vi "Main.vi"(7 "sweep rate, /min":dbl=0.2, 8 "sweep to:":dbl=4.0, 9 "sweep":T8(radio)=enum."2636a_smub") -> ()   [LabVIEW 2021]
uses:
  controls/Channel.ctl
  <instrlib>/Zurich Instruments LabOne/Public/ziTypeHandle.ctl
  controls/Measure.ctl
  controls/iPSreadCtrl.ctl
  controls/iTCreadCtrl.ctl
  controls/iPSsetCtrl.ctl
  subVIs/MFLIcommand.ctl
  controls/Source.ctl
  controls/iTCsetCtrl.ctl
  <vilib>/Utility/file.llb/Write To Spreadsheet File (DBL).vi
  <vilib>/gmath/NI_Gmath.lvlib
  <instrlib>/Keithley 2450/Keithley 2450.lvlib
  HULK SMS/SMScontrols.ctl
  <instrlib>/Zurich Instruments LabOne/Zurich Instruments LabOne.lvlib
panel:
  in  "MFLI1_AuxOut0":bool
  in  "T_Channel_sweep":i32=8
  in  "MC_RuO2":bool
  out "HandleOut 4":T1 {"Handle" format="0x%08x"; "Conn" format="0x%08x"}
  out "HandleOut 3":T1 {"Handle" format="0x%08x"; "Conn" format="0x%08x"}
  out "HandleOut 2":T1 {"Handle" format="0x%08x"; "Conn" format="0x%08x"}
  in  "MFLI4_d3":bool
  in  "MFLI4_d2":bool
  in  "MFLI4_d1":bool
  in  "MFLI4_d0":bool=TRUE
  in  "MFLI4_addr":string="DEV3532"
  in  "MFLI3_d3":bool
  in  "MFLI3_d2":bool
  in  "MFLI3_d1":bool
  in  "MFLI3_d0":bool=TRUE
  in  "MFLI3_addr":string="DEV3550"
  in  "MFLI2_d3":bool
  in  "MFLI2_d2":bool
  in  "MFLI2_d1":bool
  in  "MFLI2_d0":bool=TRUE
  in  "MFLI2_addr":string="DEV4330"
  in  "MFLI1_d3":bool
  in  "MFLI1_d2":bool
  out "HandleOut":T1 {"Handle" format="0x%08x"; "Conn" format="0x%08x"}
  in  "MFLI1_d1":bool
  in  "MFLI1_d0":bool=TRUE
  in  "MFLI1_addr":string="DEV4406"
  in  "SR830 5 oop":bool
  in  "SR830 5 ip":bool
  in  "SR830 5 addr":u8=5
  in  "SR830 4 oop":bool
  in  "SR830 4 ip":bool
  in  "SR830 3 oop":bool
  in  "SR830 3 ip":bool
  in  "SR830 2 oop":bool
  in  "SR830 2 ip":bool
  in  "SR830 1 oop":bool
  in  "SR830 1 ip":bool
  in  "SR830 4 addr":u8=4
  in  "SR830 3 addr":u8=3
  in  "SR830 2 addr":u8=2
  in  "SR830 1 addr":u8=1
  in  "MC_Cernox":bool
  in  "PT2":bool
  in  "Still":bool
  in  "Cold_Plate":bool
  in  "PT1":bool
  in  "Magnet_T":bool
  in  "2182A 4 ch2":bool
  in  "2182A 4 ch1":bool
  in  "2182A 3 ch2":bool
  in  "2182A 3 ch1":bool
  in  "2182A 2 ch2":bool
  in  "2182A 2 ch1":bool
  in  "2182A 4 addr":u8=18
  in  "2182A 3 addr":u8=17
  in  "2182A 2 addr":u8=16
  in  "2182A 1 addr":u8=15
  in  "2182A 1 ch2":bool
  in  "2182A 1 ch1":bool
  in  "Lead Chanl":T2(ring)=enum."time_sweep"
  in  "Sweep Up":bool
  in  "Stop Ramp":bool
  in  "Up Rate":dbl=0.2
  in  "Down Rate":dbl=0.2
  in  "Ramp \nUp":bool
  in  "Ramp\n Down":bool
  in  "lower limit":dbl=-4.0
  in  "upper limit":dbl=4.0
  in  "Sweep Down":bool
  in  "Stop Sweep":bool
  in  "Continuous Sweep":bool
  in  "Slave Chanl":T3=enum."b"
  in  "Double Sweep":bool
  in  "Slope":dbl
  in  "Offset":dbl
  in  "time/point, sec":dbl=1.0
  out "sweep value":dbl=2.186666666666735
  out "time delay, ms":dbl
  out "current time":timestamp=timestamp(3589630313.018 s since 1904-01-01) format="%<%H:%M:%S%1u>T"
  in  "Sweep B":bool
  out "SuperHyper":dbl=-0.4901
  in  "2461_addr_sweep":refnum<visa-resource-name>="itcetherT"
  in  "2461_meas_i":bool
  in  "2461_meas_v":bool
  out "Hyper Channel":dbl=-0.4901
  out "Sweep Channel":dbl
  out "Step Channel":dbl=-0.4901
  in  "MappingName":string
  in  "Data Folder":path=path "E:/Katya"
  out "Data file:":path=path "D:/Yanmeng/Data/Year2018/January2018/Jan2318/Jan2318x001.dat"
  in  "Initialize":bool=TRUE
  in  "Quit":bool
  in  "Refresh Time(ms)":u32=100
  in  "Monitor":bool
  in  "Linetrace or Mapping?":bool
  in  "Step and Hyerloop Setups":enum32{"Step", "HyperLoop", "SuperHyper"}(tab)
  in  "T_Channel":i32=8
  in  "Lead Chanl_step":T4(ring)=enum."2636a_smua_step" caption="Lead Chanl"
  in  "UpLimitValue":dbl
  in  "DownLimitValue":dbl
  in  "Change Sweep Range":bool
  in  "Offset_Up":dbl
  in  "Offset_Down":dbl
  in  "Slope":dbl
  in  "Down          Up":string[][](table)
  in  "Generate":bool
  in  "2461_addr_step":refnum<visa-resource-name>="itcetherT"
  in  "Channel":T3=enum."b"
  in  "Mini steps":dbl=30.0
  in  "Tolerance_Step":dbl=0.0001
  in  "Step Slope":dbl
  in  "Step Offset":dbl
  in  "diagonal step":bool
  in  "FieldRate(T/min)":dbl=0.001
  out "at field":bool
  in  "iPS _addr_step":refnum<visa-resource-name>="iPS"
  in  "step":T5(radio)=enum."time_step"
  in  "2614A_addr_step":refnum<visa-resource-name>="Keithley2614B"
  in  "2400_2_addr_step":u8=12
  in  "2400_1_addr_step":u8=12
  in  "wait between sweeps(s)":u32=1
  in  "Wait Between Step(s)":i32=1
  in  "Stop Mapping":bool
  in  "Start Mapping":bool
  in  "HyperLoop":bool
  in  "EstimateTime":bool
  out "MM:":dbl
  out "SS:":dbl
  out "HH:":dbl
  out "Finish Time":timestamp
  out "Sweep Direction":string
  out "Current Step Value":dbl
  out "Table Index":dbl
  in  "Populate step table?":bool
  in  "Step values":string[][](table)=[["-20"], ["-10"], ["-4"], ["-1"], ["3"], ["6"], ["10"], [""]]
  in  "to":dbl=1.0
  in  "step":dbl=0.001
  in  "from":dbl
  in  "SwapStepDirection":bool
  out "Hidden_HyperLoop_Swap":bool
  out "HyperLoop Hidden":bool
  in  "EstimateTime Hyper":bool
  out "MM:":dbl
  out "SS:":dbl
  out "HH:":dbl
  out "Finish Time 2":timestamp
  out "Sweep Direction 2":string
  out "Current Hyper Value":dbl
  out "HyperLoop Index":dbl
  in  "Populate HyperLoop table?":bool
  in  "HyperLoop Steps":string[][](table)=[["-20"], ["-10"], ["-4"], ["-1"], ["3"], ["6"], ["10"], [""]]
  in  "to":dbl=1.0
  in  "step":dbl=2.0
  in  "from":dbl=1.0
  in  "SuperHyper":bool
  in  "Channel_hyper":T3=enum."b"
  in  "Hyper_Mini steps":dbl=30.0
  in  "Tolerance_Hyper":dbl=0.1
  in  "Hyper Slope":dbl
  in  "Hyper Offset":dbl
  in  "diagonal_hyper":bool
  in  "Hyper_FieldRate\n(T/min)":dbl=0.1
  out "at field_hyper":bool
  in  "iPS _addr_hyper":refnum<visa-resource-name>="iPS"
  in  "iTC_addr_hyper":refnum<visa-resource-name>="iTC"
  in  "step_hyper":T6(radio)=enum."time_HyperLoop"
  in  "2336A_addr_hyper":refnum<visa-resource-name>="Keithley2614B"
  in  "2400_2_addr_hyper":u8=12
  in  "2400_1_addr_hyper":u8=12
  in  "Wait Between Hyper":i32=10
  in  "Stop HyperLoop":bool
  in  "Start HyperLoop":bool
  in  "SwapHyperDirection":bool
  out "Hidden_super_Swap":bool
  out "Super Hidden":bool
  in  "EstimateTime Hyper 2":bool
  out "MM:":dbl
  out "SS:":dbl
  out "HH:":dbl
  out "Finish Time Super":timestamp
  out "Sweep Direction3":string
  out "Current SuperHyper Value":dbl
  out "SuperHyper_Index":dbl
  in  "Populate SuperHyper table?":bool
  in  "SuperHyper Steps":string[][](table)=[["-20"], ["-10"], ["-4"], ["-1"], ["3"], ["6"], ["10"], [""]]
  in  "to":dbl=1.0
  in  "step":dbl=2.0
  in  "from":dbl=1.0
  in  "Channel_super":T3=enum."b"
  in  "Super_ministeps":dbl=30.0
  in  "Tolerance_super":dbl=0.1
  in  "Slope_super":dbl
  in  "Offset_super":dbl
  in  "diagona_super":bool
  in  "Super_FieldRate\n(T/min)":dbl=0.1
  out "at field_super":bool
  in  "iPS _addr_superhyper":refnum<visa-resource-name>="iPS"
  in  "iTC_addr_super":refnum<visa-resource-name>="iTC"
  in  "step_super":T7(radio)=enum."time_SuperHyper"
  in  "2336A_addr_super":refnum<visa-resource-name>="Keithley2614B"
  in  "2400_2_addr_super":u8=12
  in  "2400_1_addr_super":u8=12
  in  "Wait Btwn SuperHyper":i32=10
  in  "Stop SuperHyper":bool
  in  "StartSuperHyper":bool
  out "DownNameString":string
  out "UpNameString":string
  in  "Cytec_Switch":bool
  in  "Lockin_Setup":bool
  in  "TempCtrl":bool
  in  "MagnetCtrl":bool
  in  "Tolerance_Sweep":dbl=0.01
  in  "iPS_addr_sweep":refnum<visa-resource-name>="iPS"
  in  "2400 3 addr":u8=14
  in  "2400 2 addr":u8=12
  in  "2400 1 addr":u8=13
  in  "2614A addr":refnum<visa-resource-name>="TCPIP0::192.168.0.13::inst0::INSTR"
  in  "sweep":bool
  in  "MagnetField":bool
  in  "auto\nrange B":bool
  in  "measure time":bool
  in  "2636A smub meas i":bool=TRUE
  in  "2636A smub meas v":bool=TRUE
  in  "2636A smua meas i":bool
  in  "2636A smua meas v":bool
  in  "2400 3 meas i":bool
  in  "2400 2 meas i":bool
  in  "2400 2 meas v":bool
  in  "2400 3 meas v":bool
  in  "2400 1 meas i":bool
  in  "2400 1 meas v":bool
  in  "auto\nrange A":bool
  out "status 3":bool
  in  "Y_right_formula":string="brty/10/(300*10^-9)"
  in  "Yright":u16(ring)=3 caption="Y-Right:" items=["V_Sweep_AuxOut0", "2614A_smub_v", "2614A_smub_i", "time", "Magnet_Temp", "MC_RuO2_Temp", "MC_Cernox_Temp", "iTC_Step", "MFLI1_d0_x", "MFLI1_d0_y", "MFLI1_d0_freq", "MFLI1_d2_x", "MFLI1_d2_y", "MFLI1_d2_freq", "MF1_AuxOut0", "formula"]
  out "status 2":bool
  in  "Y_left_formula":string="brty/10/(300*10^-9)"
  in  "X_axis_formula":string
  in  "Yaxis":u16(ring)=3 caption="Y-Left:" items=["V_Sweep_AuxOut0", "2614A_smub_v", "2614A_smub_i", "time", "Magnet_Temp", "MC_RuO2_Temp", "MC_Cernox_Temp", "iTC_Step", "MFLI1_d0_x", "MFLI1_d0_y", "MFLI1_d0_freq", "MFLI1_d2_x", "MFLI1_d2_y", "MFLI1_d2_freq", "MF1_AuxOut0", "formula"]
  out "XY Graph":cluster{"Y Values":dbl[], "Y Values":dbl[]}[](graph)
  in  "Xaxis":u16(ring) caption="X-axis:" items=["V_Sweep_AuxOut0", "2614A_smub_v", "2614A_smub_i", "time", "Magnet_Temp", "MC_RuO2_Temp", "MC_Cernox_Temp", "iTC_Step", "MFLI1_d0_x", "MFLI1_d0_y", "MFLI1_d0_freq", "MFLI1_d2_x", "MFLI1_d2_y", "MFLI1_d2_freq", "MF1_AuxOut0", "formula"]
  out "status":bool
  in  "Show cursor":bool
  in  "Hulk_B_meas (Vnano)":bool
  in  "Hulk_SMS_addr":refnum<visa-resource-name>="TCPIP0::10.99.75.17::inst0::INSTR"
  in  "formula_variables":string[](array[string])=["a", "b", "c", "d", "e", "e", "f", "g", "h", "i", "j"]
  out "data":dbl[](array[numeric])
  out "Figure_axis":string[](array[string])=["HULK_SMS_output", "SR830_1_ip", "SR830_1_oop"]
  out "data_caption":string="HULK_SMS_output\tSR830_1_ip\tSR830_1_oop\t"
  # "Current Value of Sweep and Step Channels"
  # "Sweep Channel Setup"
  # "SweepChannel"
  # "address"
  # "2400_1"
  # "2400_2"
  # "2400_3"
  # "2614A_smua"
  # "2614A_smub"
  # "time"
  # "Triton B"
  # "MC_Temp"
  # "2450_1"
  # "MF1 AuxOut0"
  # "sweep"
  # "!Current sweep!"
  # "MagnetField"
  # "measure"
  # "voltage (_v)"
  # "current (_i)"
  # "blue"
  # "red"
  # "Measure Channels"
  # "MFLI Lock-in amplifiers"
  # "SRS Lock-in amplifiers"
  # "address"
  # "SR830_1"
  # "SR830_2"
  # "SR830_3"
  # "SR830_4"
  # "d0"
  # "measure"
  # "SR830_5"
  # "d1"
  # "in phase (_ip)"
  # "d2"
  # "out of phase (_oop)"
  # "d3"
  # "Nanovoltmeters"
  # "Temperature"
  # "address"
  # "Dilution Circuit"
  # "PulseTube"
  # "MC_RuO2"
  # "measure"
  # "2182A_1"
  # "2182A_2"
  # "2182A_3"
  # "2182A_4"
  # "channel 1 (_ch1)"
  # "channel 2 (_ch2)"
  # "(not recommended, slow)"
  # "Sweep Parameters Setup"
  # "Up"
  # "Down"
  # "Limits"
  # "Rate\n(/min)"
  # "Step Channel Setup"
  # "StepChannel"
  # "addres"
  # "Triton B"
  # "Triton T"
  # "2400_1"
  # "2400_2"
  # "2636A_smua"
  # "2636A_smub"
  # "time"
  # "2461"
  # "step"
  # "Step Table"
  # "Step Table"
  # "Hyper Loop Setup"
  # "StepChannel"
  # "addres"
  # "2400_1"
  # "2400_2"
  # "2636A_smua"
  # "2636A_smub"
  # "time"
  # "Teslatron iPS"
  # "Teslatron iTC"
  # "step"
  # "SuperHyper Setup"
  # "StepChannel"
  # "addres"
  # "Teslatron iPS"
  # "Teslatron iTC"
  # "2400_1"
  # "2400_2"
  # "2636A_smua"
  # "2636A_smub"
  # "time"
  # "step"
  # "Step Table"
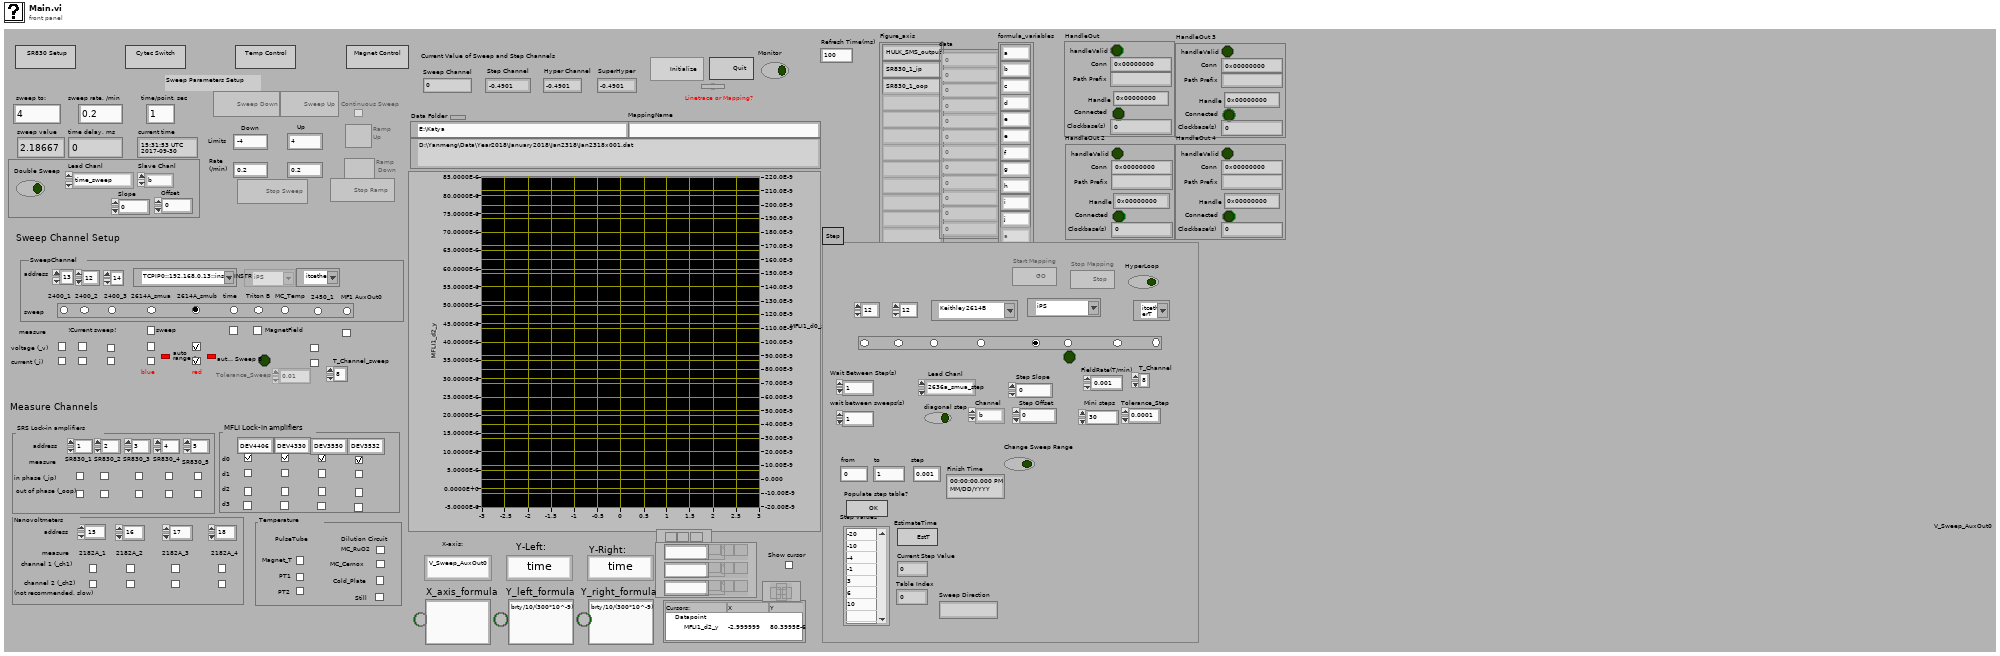
[diagram p1: front panel]
types:
  T1 = typedef "Zurich Instruments LabOne.lvlib/ziTypeHandle.ctl" = cluster{"handleValid":bool, "Conn":u64, "Path Prefix":string, "Handle":u64, "Connected":bool, "Clockbase(s)":dbl}
  T2 = enum16{"2400_1", "2400_2", "2400_3", "2636a_smua", "2636a_smub", "time_sweep", "iPS", "iTC", "2461"}
  T3 = typedef "Channel.ctl" = enum16{"a", "b"}
  T4 = enum16{"V2400_1_step", "V2400_2_step", "2636a_smua_step", "2636a_smub_step", "time_step", "iPS_step", "iTC_step", "2461_Curr"}
  T5 = enum32{"V2400_1_Step", "V2400_2_step", "2636_smua_step", "2636_smub_step", "time_step", "iTC_step", "iPS_step", "2461_Curr"}
  T6 = enum32{"2400_1_HyperLoop", "2400_2_HyperLoop", "2636_smua_HyperLoop", "2636_smub_HyperLoop", "time_HyperLoop", "iTC_HyperLoop", "iPS_HyperLoop"}
  T7 = enum32{"2400_1_SuperHyper", "2400_2_SuperHyper", "2636_smua_SuperHyper", "2636_smub_SuperHyper", "time_SuperHyper", "iTC_SuperHyper", "iPS_SuperHyper"}
  T8 = enum32{"2400_1", "2400_2", "2400_3", "2636a_smua", "2636a_smub", "time_sweep", "iPS", "iTC", "2461", "AuxOut0"}
  T9 = cluster{"vi reference":refnum<vi>, "vi reference":refnum<vi>}
  T10 = enum8{"Enabled", "Disabled", "Disabled and Grayed Out"}
  T11 = typedef "Measure.ctl" = enum16{"Voltage", "Current", "Resistance", "Power"}
  T12 = typedef "SMScontrols.ctl" = enum16{"UPDATE", "GET OUTPUT", "RAMP ZERO", "RAMP MID", "RAMP MAX", "RAMP STATUS", "PAUSE OFF", "PAUSE ON", "HEATER OFF", "HEATER ON", "TESLA OFF", "TESLA ON", "DIRECTION +", "DIRECTION -", "DIRECTION 0", "SET MID", "SET MAX", "SET RAMP", "SET LIMIT", "SET TPA", "SET HEATER"}
  T13 = typedef "iPSreadCtrl.ctl" = enum16{"OutputField", "MagnetField", "Switch Heater Temp", "Field Rate", "Magnet Temp", "OutputVoltage"}
  T14 = typedef "iTCreadCtrl.ctl" = enum16{"PT1 Temp", "PT2 Temp", "Sample Temp", "VTI Temp", "Needle Valve", "VTI Heater Power", "Sample Heater Power", "VTI Pressure"}
  T15 = typedef "MFLIcommand.ctl" = enum16{"initialise", "measure XY on demod0", "measure XY on demod1", "measure XY on demod2", "measure XY on demod3", "Set AuxOut0", "Set AuxOut1", "Set AuxOut2", "Set AuxOut3", "Get AuxOut0", "Set Osc0 Ampl", "Set Osc1 Ampl", "Set Osc0 Freq", "Set Osc1 Freq", "SigIns Autorange", "finalise"}
  T16 = typedef "iPSsetCtrl.ctl" = enum16{"Set Target Field", "Set Target Field Rate", "Switch Heater ON", "Switch Heater OFF", "Go to Field", "Go to Zero", "Hold"}
  T17 = enum32{"Radio Selection 1", "Radio Selection 2", "Radio Selection 3", "Radio Selection 4", "Radio Selection 5", "Radio Selection 6", "Radio Selection 7"}
  T18 = typedef "Source.ctl" = enum16{"Current", "Voltage"}
  T19 = typedef "iTCsetCtrl.ctl" = enum16{"Set Sample Temp", "Set VTI Temp", "Set Needle Valve", "Set VTI Heater Power", "Set Sample Heater Power", "Set VTI Pressure"}
  T20 = typedef "Zurich Instruments LabOne.lvlib/ziTypeDemodSampleSingle.ctl" = cluster{"Timestamps (ticks)":u64, "X (Vrms)":dbl, "Y (Vrms)":dbl, "Osc Phase (deg)":dbl, "Freq (Hz)":dbl, "DIO":u32, "AuxIn0 (V)":dbl, "AuxIn1 (V)":dbl, "Trigger":u32}
  T21 = cluster{"handleValid":bool, "Conn":u64, "Path Prefix":string, "Handle":u64, "Connected":bool, "Clockbase(s)":dbl}
  T22 = enum32{"Bad", "Idle", "Run top level", "Running"}
diagram:
  # "This template is for the Producer/Consumer design pattern."
  # "initial value"
  n1 = flat-sequence {
    tunnel: [w15] -> w2
    tunnel: [w7] -> w1
    frame #0 {
      n2 = Current VI's Path() -> (path=w22:path)
      n3 = Strip Path(path=w22) -> (stripped path=w13:path)  [unwired: 1 out]
      n4 = Build Path(base path=w13, name or relative path="subVIs\\MagnetControl.vi") -> (appended path=w18:path)
      n5 = Build Path(base path=w13, name or relative path="subVIs\\TemperatureControl.vi") -> (appended path=w19:path)
      n6 = Build Path(base path=w13, name or relative path="subVIs\\CytecControl.vi") -> (appended path=w11:path)
      n7 = Build Path(base path=w13, name or relative path="subVIs\\Lockin Control Panel.vi") -> (appended path=w10:path)
      n8 = Open VI Reference(vi path=w18) -> (vi reference=w16:refnum<vi>)  [unwired: 5 in, 1 out]
      n9 = Open VI Reference(vi path=w19) -> (vi reference=w17:refnum<vi>)  [unwired: 5 in, 1 out]
      n10 = Open VI Reference(vi path=w10) -> (vi reference=w8:refnum<vi>)  [unwired: 5 in, 1 out]
      n11 = Open VI Reference(vi path=w11) -> (vi reference=w9:refnum<vi>)  [unwired: 5 in, 1 out]
      n12 = Bundle("vi reference"=w9, "vi reference"=w8) -> (w7:T9)  [unwired: 1 in]
      n13 = Bundle("vi reference"=w17, "vi reference"=w16) -> (w15:T9)  [unwired: 1 in]
    }
    frame #1 {
      w24 = T10."Disabled and Grayed Out" ("Disabled")
      w26 = T10."Enabled" ("Disabled")
      # "1 = 2400 1\n2 = 2400 2\n3 = 2400 3\n4 = 2636a smua\n5 = 2636a smub\n6 = do not sweep, just time\n7 = Magnetic Field IPS120\n8= 2461 smu"
      # "delete previous values"
      n14 = property on="Linetrace or Mapping?" class="Bool (strict)"() -> ("Value"=w25:bool)  [unwired: 2 in, 2 out]
      n15 = case shown="True" w25 {
        frame False {
          w29 = FALSE ("Change Sweep Range")
          w35 = FALSE ("Visible")
          w30 = FALSE ("HyperLoop")
          w36 = T10."Disabled and Grayed Out" ("Disabled")
          w42 = T10."Enabled" ("Disabled")
          n16 = property on="UpLimitValue" class="DigNum (strict)"("Visible"=w35) -> ()  [unwired: 2 in, 2 out]
          n17 = property on="DownLimitValue" class="DigNum (strict)"("Visible"=w35) -> ()  [unwired: 2 in, 2 out]
          n18 = property on="Generate" class="Bool"("Visible"=w35) -> ()  [unwired: 2 in, 2 out]
          n19 = property on="Offset_Up" class="DigNum (strict)"("Visible"=w35) -> ()  [unwired: 2 in, 2 out]
          n20 = property on="Down          Up" class="Tbl (strict)"("Visible"=w35) -> ()  [unwired: 2 in, 2 out]
          n21 = property on="Slope" class="DigNum (strict)"("Visible"=w35) -> ()  [unwired: 2 in, 2 out]
          n22 = property on="Offset_Down" class="DigNum (strict)"("Visible"=w35) -> ()  [unwired: 2 in, 2 out]
          n23 = property on="Change Sweep Range" class="Bool (strict)"("Value"=w29) -> ()  [unwired: 2 in, 2 out]
          n24 = property on="SwapHyperDirection" class="Bool (strict)"("Value"=w29) -> ()  [unwired: 2 in, 2 out]
          n25 = property on="Tolerance_Sweep" class="DigNum (strict)"("DisabledEnum"=w42) -> ()  [unwired: 2 in, 2 out]
          n26 = property on="Ramp\n Down" class="Bool"("DisabledEnum"=w42) -> ()  [unwired: 2 in, 2 out]
          n27 = property on="sweep" class="RadioBtnsControl (strict)"("DisabledEnum"=w42) -> ()  [unwired: 2 in, 2 out]
          n28 = property on="2182A 1 addr" class="DigNum (strict)"("DisabledEnum"=w42) -> ()  [unwired: 2 in, 2 out]
          n29 = property on="2182A 2 addr" class="DigNum (strict)"("DisabledEnum"=w42) -> ()  [unwired: 2 in, 2 out]
          n30 = property on="2182A 3 addr" class="DigNum (strict)"("DisabledEnum"=w42) -> ()  [unwired: 2 in, 2 out]
          n31 = property on="2182A 4 addr" class="DigNum (strict)"("DisabledEnum"=w42) -> ()  [unwired: 2 in, 2 out]
          n32 = property on="2400 1 addr" class="DigNum (strict)"("DisabledEnum"=w42) -> ()  [unwired: 2 in, 2 out]
          n33 = property on="Continuous Sweep" class="Bool (strict)"("DisabledEnum"=w42) -> ()  [unwired: 2 in, 2 out]
          n34 = property on="Sweep Down" class="Bool"("DisabledEnum"=w42) -> ()  [unwired: 2 in, 2 out]
          n35 = property on="Sweep Up" class="Bool"("DisabledEnum"=w42) -> ()  [unwired: 2 in, 2 out]
          n36 = property on="SR830 2 addr" class="DigNum (strict)"("DisabledEnum"=w42) -> ()  [unwired: 2 in, 2 out]
          n37 = property on="SR830 3 addr" class="DigNum (strict)"("DisabledEnum"=w42) -> ()  [unwired: 2 in, 2 out]
          n38 = property on="2400 2 addr" class="DigNum (strict)"("DisabledEnum"=w42) -> ()  [unwired: 2 in, 2 out]
          n39 = property on="2400 3 addr" class="DigNum (strict)"("DisabledEnum"=w42) -> ()  [unwired: 2 in, 2 out]
          n40 = property on="2614A addr" class="VISAName"("DisabledEnum"=w42) -> ()  [unwired: 2 in, 2 out]
          n41 = property on="SR830 1 addr" class="DigNum (strict)"("DisabledEnum"=w42) -> ()  [unwired: 2 in, 2 out]
          n42 = property on="SR830 4 addr" class="DigNum (strict)"("DisabledEnum"=w42) -> ()  [unwired: 2 in, 2 out]
          n43 = property on="Ramp \nUp" class="Bool"("DisabledEnum"=w42) -> ()  [unwired: 2 in, 2 out]
          n44 = property on="Step and Hyerloop Setups" class="TabCtl (strict)"() -> ("Pages"=w31:refnum<vi>[])  [unwired: 2 in, 2 out]
          n45 = property on="Step and Hyerloop Setups" class="TabCtl (strict)"() -> ("Pages"=w40:refnum<vi>[])  [unwired: 2 in, 2 out]
          n46 = Index Array(array=w31, index=2) -> (element=w32:refnum<vi>)
          n47 = Index Array(array=w40, index=1) -> (element=w39:refnum<vi>)
          n48 = property class="Page"(reference=w32, "PageVis"=FALSE ("Page Visible")) -> ()  [unwired: 1 in, 2 out]
          n49 = property class="Page"(reference=w39, "PageVis"=FALSE ("Page Visible")) -> ()  [unwired: 1 in, 2 out]
          n50 = property on="HyperLoop" class="Bool (strict)"("Value"=w30) -> ()  [unwired: 2 in, 2 out]
          n51 = property on="SuperHyper" class="Bool (strict)"("Value"=w30) -> ()  [unwired: 2 in, 2 out]
          n52 = property on="MappingName" class="Str"("Visible"=FALSE) -> ()  [unwired: 2 in, 2 out]
          n53 = property on="step" class="RadioBtnsControl (strict)"("DisabledEnum"=w36) -> ()  [unwired: 2 in, 2 out]
          n54 = property on="diagonal step" class="Bool (strict)"("DisabledEnum"=w36) -> ()  [unwired: 2 in, 2 out]
          n55 = property on="FieldRate(T/min)" class="DigNum (strict)"("DisabledEnum"=w36) -> ()  [unwired: 2 in, 2 out]
          n56 = property on="Step Offset" class="DigNum (strict)"("DisabledEnum"=w36) -> ()  [unwired: 2 in, 2 out]
          n57 = property on="Tolerance_Step" class="DigNum (strict)"("DisabledEnum"=w36) -> ()  [unwired: 2 in, 2 out]
          n58 = property on="Step Slope" class="DigNum (strict)"("DisabledEnum"=w36) -> ()  [unwired: 2 in, 2 out]
          n59 = property on="iPS _addr_step" class="VISAName"("DisabledEnum"=w36) -> ()  [unwired: 2 in, 2 out]
          n60 = property on="wait between sweeps(s)" class="DigNum (strict)"("DisabledEnum"=w36) -> ()  [unwired: 2 in, 2 out]
          n61 = property on="2614A_addr_step" class="VISAName"("DisabledEnum"=w36) -> ()  [unwired: 2 in, 2 out]
          n62 = property on="Start Mapping" class="Bool"("DisabledEnum"=w36) -> ()  [unwired: 2 in, 2 out]
          n63 = property on="2400_1_addr_step" class="DigNum (strict)"("DisabledEnum"=w36) -> ()  [unwired: 2 in, 2 out]
          n64 = property on="Wait Between Step(s)" class="DigNum (strict)"("DisabledEnum"=w36) -> ()  [unwired: 2 in, 2 out]
          n65 = property on="2400_2_addr_step" class="DigNum (strict)"("DisabledEnum"=w36) -> ()  [unwired: 2 in, 2 out]
          n66 = property on="HyperLoop" class="Bool (strict)"("DisabledEnum"=w36) -> ()  [unwired: 2 in, 2 out]
        }
        frame True {
          w43 = FALSE ("Change Sweep Range")
          w49 = FALSE ("Visible")
          w44 = FALSE ("HyperLoop")
          w56 = T10."Disabled and Grayed Out" ("Disabled")
          w50 = T10."Enabled" ("Disabled")
          n67 = property on="UpLimitValue" class="DigNum (strict)"("Visible"=w49) -> ()  [unwired: 2 in, 2 out]
          n68 = property on="DownLimitValue" class="DigNum (strict)"("Visible"=w49) -> ()  [unwired: 2 in, 2 out]
          n69 = property on="Generate" class="Bool"("Visible"=w49) -> ()  [unwired: 2 in, 2 out]
          n70 = property on="Offset_Up" class="DigNum (strict)"("Visible"=w49) -> ()  [unwired: 2 in, 2 out]
          n71 = property on="Down          Up" class="Tbl (strict)"("Visible"=w49) -> ()  [unwired: 2 in, 2 out]
          n72 = property on="Slope" class="DigNum (strict)"("Visible"=w49) -> ()  [unwired: 2 in, 2 out]
          n73 = property on="Offset_Down" class="DigNum (strict)"("Visible"=w49) -> ()  [unwired: 2 in, 2 out]
          n74 = property on="SwapHyperDirection" class="Bool (strict)"("Value"=w43) -> ()  [unwired: 2 in, 2 out]
          n75 = property on="Change Sweep Range" class="Bool (strict)"("Value"=w43) -> ()  [unwired: 2 in, 2 out]
          n76 = property on="Ramp\n Down" class="Bool"("DisabledEnum"=w56) -> ()  [unwired: 2 in, 2 out]
          n77 = property on="sweep" class="RadioBtnsControl (strict)"("DisabledEnum"=w56) -> ()  [unwired: 2 in, 2 out]
          n78 = property on="2182A 1 addr" class="DigNum (strict)"("DisabledEnum"=w56) -> ()  [unwired: 2 in, 2 out]
          n79 = property on="2182A 2 addr" class="DigNum (strict)"("DisabledEnum"=w56) -> ()  [unwired: 2 in, 2 out]
          n80 = property on="2182A 3 addr" class="DigNum (strict)"("DisabledEnum"=w56) -> ()  [unwired: 2 in, 2 out]
          n81 = property on="2182A 4 addr" class="DigNum (strict)"("DisabledEnum"=w56) -> ()  [unwired: 2 in, 2 out]
          n82 = property on="2400 1 addr" class="DigNum (strict)"("DisabledEnum"=w56) -> ()  [unwired: 2 in, 2 out]
          n83 = property on="Tolerance_Sweep" class="DigNum (strict)"("DisabledEnum"=w56) -> ()  [unwired: 2 in, 2 out]
          n84 = property on="Sweep Down" class="Bool"("DisabledEnum"=w56) -> ()  [unwired: 2 in, 2 out]
          n85 = property on="SR830 2 addr" class="DigNum (strict)"("DisabledEnum"=w56) -> ()  [unwired: 2 in, 2 out]
          n86 = property on="SR830 3 addr" class="DigNum (strict)"("DisabledEnum"=w56) -> ()  [unwired: 2 in, 2 out]
          n87 = property on="2400 2 addr" class="DigNum (strict)"("DisabledEnum"=w56) -> ()  [unwired: 2 in, 2 out]
          n88 = property on="2400 3 addr" class="DigNum (strict)"("DisabledEnum"=w56) -> ()  [unwired: 2 in, 2 out]
          n89 = property on="2614A addr" class="VISAName"("DisabledEnum"=w56) -> ()  [unwired: 2 in, 2 out]
          n90 = property on="SR830 1 addr" class="DigNum (strict)"("DisabledEnum"=w56) -> ()  [unwired: 2 in, 2 out]
          n91 = property on="SR830 4 addr" class="DigNum (strict)"("DisabledEnum"=w56) -> ()  [unwired: 2 in, 2 out]
          n92 = property on="Ramp \nUp" class="Bool"("DisabledEnum"=w56) -> ()  [unwired: 2 in, 2 out]
          n93 = property on="Step and Hyerloop Setups" class="TabCtl (strict)"() -> ("Pages"=w45:refnum<vi>[])  [unwired: 2 in, 2 out]
          n94 = property on="Step and Hyerloop Setups" class="TabCtl (strict)"() -> ("Pages"=w54:refnum<vi>[])  [unwired: 2 in, 2 out]
          n95 = property on="Continuous Sweep" class="Bool (strict)"("DisabledEnum"=w56) -> ()  [unwired: 2 in, 2 out]
          n96 = property on="Continuous Sweep" class="Bool (strict)"("Value"=FALSE ("Continuous Sweep")) -> ()  [unwired: 2 in, 2 out]
          n97 = Index Array(array=w45, index=2) -> (element=w46:refnum<vi>)
          n98 = Index Array(array=w54, index=1) -> (element=w53:refnum<vi>)
          n99 = property class="Page"(reference=w46, "PageVis"=FALSE ("Page Visible")) -> ()  [unwired: 1 in, 2 out]
          n100 = property on="SuperHyper" class="Bool (strict)"("Value"=w44) -> ()  [unwired: 2 in, 2 out]
          n101 = property class="Page"(reference=w53, "PageVis"=FALSE ("Page Visible")) -> ()  [unwired: 1 in, 2 out]
          n102 = property on="HyperLoop" class="Bool (strict)"("Value"=w44) -> ()  [unwired: 2 in, 2 out]
          n103 = property on="MappingName" class="Str"("Visible"=TRUE) -> ()  [unwired: 2 in, 2 out]
          n104 = property on="step" class="RadioBtnsControl (strict)"("DisabledEnum"=w50) -> ()  [unwired: 2 in, 2 out]
          n105 = property on="Step Offset" class="DigNum (strict)"("DisabledEnum"=w50) -> ()  [unwired: 2 in, 2 out]
          n106 = property on="diagonal step" class="Bool (strict)"("DisabledEnum"=w50) -> ()  [unwired: 2 in, 2 out]
          n107 = property on="Step Slope" class="DigNum (strict)"("DisabledEnum"=w50) -> ()  [unwired: 2 in, 2 out]
          n108 = property on="iPS _addr_step" class="VISAName"("DisabledEnum"=w50) -> ()  [unwired: 2 in, 2 out]
          n109 = property on="wait between sweeps(s)" class="DigNum (strict)"("DisabledEnum"=w50) -> ()  [unwired: 2 in, 2 out]
          n110 = property on="FieldRate(T/min)" class="DigNum (strict)"("DisabledEnum"=w50) -> ()  [unwired: 2 in, 2 out]
          n111 = property on="2614A_addr_step" class="VISAName"("DisabledEnum"=w50) -> ()  [unwired: 2 in, 2 out]
          n112 = property on="Start Mapping" class="Bool"("DisabledEnum"=w50) -> ()  [unwired: 2 in, 2 out]
          n113 = property on="2400_1_addr_step" class="DigNum (strict)"("DisabledEnum"=w50) -> ()  [unwired: 2 in, 2 out]
          n114 = property on="Wait Between Step(s)" class="DigNum (strict)"("DisabledEnum"=w50) -> ()  [unwired: 2 in, 2 out]
          n115 = property on="Tolerance_Step" class="DigNum (strict)"("DisabledEnum"=w50) -> ()  [unwired: 2 in, 2 out]
          n116 = property on="2400_2_addr_step" class="DigNum (strict)"("DisabledEnum"=w50) -> ()  [unwired: 2 in, 2 out]
          n117 = property on="HyperLoop" class="Bool (strict)"("DisabledEnum"=w50) -> ()  [unwired: 2 in, 2 out]
        }
      }
      n118 = property on="time delay, ms" class="DigNum (strict)"("Value"=u32 0 ("delib time delay")) -> ()  [unwired: 2 in, 2 out]
      n119 = local write "data"(dbl[] [] ("data")) -> ()
      n120 = property on="Monitor" class="Bool (strict)"() -> ("Value"=w23:bool)  [unwired: 2 in, 2 out]
      n121 = property on="formula_variables" class="Arr (strict)"("Visible"=w23) -> ()  [unwired: 2 in, 2 out]
      n122 = property on="data" class="Arr (strict)"("Visible"=w23) -> ()  [unwired: 2 in, 2 out]
      n123 = property on="Figure_axis" class="Arr (strict)"("Visible"=w23) -> ()  [unwired: 2 in, 2 out]
      n124 = property on="Stop Mapping" class="Bool"("DisabledEnum"=w24) -> ()  [unwired: 2 in, 2 out]
      n125 = property on="Stop Sweep" class="Bool"("DisabledEnum"=w24) -> ()  [unwired: 2 in, 2 out]
      n126 = property on="Stop Ramp" class="Bool"("DisabledEnum"=w24) -> ()  [unwired: 2 in, 2 out]
      n127 = property on="sweep" class="RadioBtnsControl (strict)"("DisabledEnum"=w26) -> ()  [unwired: 2 in, 2 out]
      n128 = property on="2182A 1 addr" class="DigNum (strict)"("DisabledEnum"=w26) -> ()  [unwired: 2 in, 2 out]
      n129 = property on="2182A 2 addr" class="DigNum (strict)"("DisabledEnum"=w26) -> ()  [unwired: 2 in, 2 out]
      n130 = property on="2182A 3 addr" class="DigNum (strict)"("DisabledEnum"=w26) -> ()  [unwired: 2 in, 2 out]
      n131 = property on="2182A 4 addr" class="DigNum (strict)"("DisabledEnum"=w26) -> ()  [unwired: 2 in, 2 out]
      n132 = property on="2400 1 addr" class="DigNum (strict)"("DisabledEnum"=w26) -> ()  [unwired: 2 in, 2 out]
      n133 = property on="SR830 2 addr" class="DigNum (strict)"("DisabledEnum"=w26) -> ()  [unwired: 2 in, 2 out]
      n134 = property on="SR830 3 addr" class="DigNum (strict)"("DisabledEnum"=w26) -> ()  [unwired: 2 in, 2 out]
      n135 = property on="2400 2 addr" class="DigNum (strict)"("DisabledEnum"=w26) -> ()  [unwired: 2 in, 2 out]
      n136 = property on="2400 3 addr" class="DigNum (strict)"("DisabledEnum"=w26) -> ()  [unwired: 2 in, 2 out]
      n137 = property on="2614A addr" class="VISAName"("DisabledEnum"=w26) -> ()  [unwired: 2 in, 2 out]
      n138 = property on="SR830 1 addr" class="DigNum (strict)"("DisabledEnum"=w26) -> ()  [unwired: 2 in, 2 out]
      n139 = property on="SR830 4 addr" class="DigNum (strict)"("DisabledEnum"=w26) -> ()  [unwired: 2 in, 2 out]
    }
  }
  n140 = Obtain Queue(name (unnamed)="Action", element data type="" ("data (can be any type)")) -> (queue out=w3:refnum<queue>)  [unwired: 3 in, 2 out]
  n141 = while {
    tunnel: [w60] -> w4
    tunnel: w3 -> [w58]
    stop <- w59 stop-if-true
    # "This loop is a consumer loop."
    n142 = Dequeue Element(queue=w58) -> (queue out=w60:refnum<queue>, element=w61:string)  [unwired: 2 in, 2 out]
    n143 = case shown="\"Step to Next Value\"" w61 {
      tunnel: w60 -> [w62 _ _ _ w5322 w5579 w5799 _]
      tunnel: w60 -> [_ _ w1360 w3554 _ _ _ _]
      tunnel: [_ _ _ _ _ _ _ TRUE] -> w59
      frame "Idle", Default {
        # "0 = SR830_1_ip\n1 = SR830_1_oop\n2 = SR830_2_ip\n3 = SR830_2_oop\n4 = SR830_3_ip\n5 = SR830_3_oop\n6 = SR830_4_ip \n7 = SR830_4_oop \n8 = SR830_5_ip \n9 = SR830_5_oop \n10= 2400_1_v \n11= 2400_1_i \n12 = 2400_2_v\n13 = 2400_2_i \n14 = 2400_3_v \n15 = 2400_3_i \n16 = 2182A_1_ch1 \n17 = 2182A_1_ch2 \n18 = 2182A_2_ch1 \n19 = 2182A_2_ch2\n20 = 2182A_3_ch1 \n21 = 2182A_3_ch2 \n22 = 2182A_4_ch1 \n23 = 2182A_4_ch2 \n24 = 2636A_smua_v \n25 = 2636A_smua_i \n26 = 2636A_smub_v \n27 = 2636A_smub_i \n28 = time\n29 = iPS_Field\n30 = iPS_Magnet_T\n31 = iPS__SH_T\n32 = iTC _sample_T\n33 = iTC _VTI_T\n34 = iTC _PT1_T\n35 = iTC _PT2_T\n36 = iTC _VTI_P\n37 = 2461_meas_v\n38= 2461_meas_i\n39= Step_Value\n40= HyperLoop_Step\n41= SuperHyper_Step"
        n144 = stacked-sequence {
          tunnel: w62 -> [_ _ _ _ w1356]
          frame #0 {
            # "Read current value of sweep channel"
            # "1 = 2400 1\n2 = 2400 2\n3 = 2400 3\n4 = 2636a smua\n5 = 2636a smub\n6 = do not sweep, just time\n7 =IPS120-10\n8 =2461_smu"
            n145 = property on="sweep" class="RadioBtnsControl (strict)"() -> ("Value"=w64:T8)  [unwired: 2 in, 2 out]
            n146 = case "reads current value from instrument which will be sweeping" shown="\"AuxOut0\"" w64 {
              tunnel: [w65 w75 w84 w93 w97 0.0 ("Measuremet") w102 w182 w197] -> w63
              frame "2400_1", Default {
                # "reads the voltage on 2400 1"
                n147 = local read "2400 1 addr"() -> (w69:u8)
                n148 = Number To Decimal String(number=w69) -> (decimal integer string=w70:string)  [unwired: 1 in]
                n149 = GPIB Write(0:w70, 1:":READ?") -> (6:w66:errorcluster)  [unwired: 3 in, 1 out]
                n150 = GPIB Read(0:w70, 1:3200, 3:w66) -> (5:w72:string)  [unwired: 2 in, 2 out]
                n151 = String Subset(string=w72, length (rest)=13) -> (substring=w73:string)  [unwired: 1 in]
                n152 = Fract/Exp String To Number(string=w73) -> (number=w65:dbl)  [unwired: 3 in, 1 out]
              }
              frame "2400_2" {
                # "reads the current on 2400 2"
                n153 = local read "2400 2 addr"() -> (w79:u8)
                n154 = Number To Decimal String(number=w79) -> (decimal integer string=w80:string)  [unwired: 1 in]
                n155 = GPIB Write(0:w80, 1:":READ?") -> (6:w76:errorcluster)  [unwired: 3 in, 1 out]
                n156 = GPIB Read(0:w80, 1:3200, 3:w76) -> (5:w82:string)  [unwired: 2 in, 2 out]
                n157 = String Subset(string=w82, offset (0)=14, length (rest)=13) -> (substring=w83:string)
                n158 = Fract/Exp String To Number(string=w83) -> (number=w75:dbl)  [unwired: 3 in, 1 out]
              }
              frame "2400_3" {
                # "reads the voltage on 2400 3"
                n159 = local read "2400 3 addr"() -> (w88:u8)
                n160 = Number To Decimal String(number=w88) -> (decimal integer string=w89:string)  [unwired: 1 in]
                n161 = GPIB Write(0:w89, 1:":READ?") -> (6:w85:errorcluster)  [unwired: 3 in, 1 out]
                n162 = GPIB Read(0:w89, 1:3200, 3:w85) -> (5:w91:string)  [unwired: 2 in, 2 out]
                n163 = String Subset(string=w91, length (rest)=13) -> (substring=w92:string)  [unwired: 1 in]
                n164 = Fract/Exp String To Number(string=w92) -> (number=w84:dbl)  [unwired: 3 in, 1 out]
              }
              frame "2636a_smua" {
                # "reads the voltage on 2636a smua"
                n165 = local read "2614A addr"() -> (w96:refnum<visa-resource-name>)
                n166 = call "SinglePointMeasurement.vi"("Measure"=Measure."Voltage", "Channel"=Channel."a", "VISA resource name 2"=w96) -> ("Measuremet"=w93:dbl)  [unwired: 3 in, 4 out]
              }
              frame "2636a_smub" {
                # "reads the voltage on 2636a smub"
                n167 = local read "2614A addr"() -> (w100:refnum<visa-resource-name>)
                n168 = call "SinglePointMeasurement.vi"("Measure"=Measure."Voltage", "Channel"=Channel."b", "VISA resource name 2"=w100) -> ("Measuremet"=w97:dbl)  [unwired: 3 in, 4 out]
              }
              frame "time_sweep" {
              }
              frame "iPS" {
                n169 = disable-structure shown="Enabled" {
                  disable-tunnel: [w103 w180] -> w102
                  frame Disabled {
                    n170 = stacked-sequence {
                      tunnel: [_ _ _ _ _ _ _ w161 _] -> w103
                      frame #0 {
                        # "initialize interface of HULK SMS"
                        n171 = local read "Hulk_SMS_addr"() -> (w110:refnum<visa-resource-name>)
                        n172 = VISA Open(VISA resource name=w110) -> (VISA resource name=w109:refnum<visa-resource-name>, error out=w108:errorcluster)  [unwired: 4 in]
                        n173 = VISA Clear(VISA resource name=w109, error in (no error)=w108) -> (VISA resource name out=w106:refnum<visa-resource-name>, error out=w105:errorcluster)
                        n174 = property class="Instr"(reference=w106, error in=w105, "General Settings:Timeout Value"=u32 2000) -> (error out=w104:errorcluster)  [unwired: 1 out]
                        n175 = local write item#-1(w104) -> ()
                      }
                      frame #1 {
                        w111 = SMScontrols."UPDATE" ("SMS controls")
                        # "check intialization"
                        n176 = local read "Hulk_SMS_addr"() -> (w115:refnum<visa-resource-name>)
                        n177 = local read item#-1() -> (w114)
                        n178 = call "SMSsendCommand.vi"("HULK SMS address in"=w115, "SMS controls"=w111, "error in"=w114) -> ("HULK SMS address out"=w116:refnum<visa-resource-name>, "error out"=w117:errorcluster)  [unwired: 14 in, 1 out]
                        n179 = call "WaitRS232.vi"("error in"=w117, "delay[160 ms]"=u32 1000) -> ("error out"=w119:errorcluster)  [unwired: 1 in]
                        n180 = call "SMSread.vi"("HULK SMS address in"=w116, "SMS controls"=w111, "error in"=w119) -> ("read buffer"=w112:string, "error out"=w113:errorcluster)  [unwired: 11 in, 4 out]
                        n181 = local write item#-1(w112) -> ()
                        n182 = local write item#-1(w113) -> ()
                      }
                      frame #2 {
                        n183 = Wait (ms)(milliseconds to wait=u32 200) -> ()  [unwired: 1 out]
                      }
                      frame #3 {
                        w121 = SMScontrols."TESLA ON" ("SMS controls")
                        # "set units to tesla"
                        n184 = local read "Hulk_SMS_addr"() -> (w125:refnum<visa-resource-name>)
                        n185 = local read item#-1() -> (w124)
                        n186 = call "SMSsendCommand.vi"("HULK SMS address in"=w125, "SMS controls"=w121, "error in"=w124) -> ("HULK SMS address out"=w126:refnum<visa-resource-name>, "error out"=w127:errorcluster)  [unwired: 14 in, 1 out]
                        n187 = call "WaitRS232.vi"("error in"=w127, "delay[160 ms]"=u32 1000) -> ("error out"=w129:errorcluster)  [unwired: 1 in]
                        n188 = call "SMSread.vi"("HULK SMS address in"=w126, "SMS controls"=w121, "error in"=w129) -> ("read buffer"=w122:string, "error out"=w123:errorcluster)  [unwired: 11 in, 4 out]
                        n189 = local write item#-1(w122) -> ()
                        n190 = local write item#-1(w123) -> ()
                      }
                      frame #4 {
                        w130 = T10."Disabled and Grayed Out" ("Disabled")
                        # "sorry, no control of sweep rate and target\nvalue during sweeping\n\n!!! do not forget to reactivate it in the PAUSE mode!!!"
                      }
                      frame #5 {
                        w134 = SMScontrols."SET RAMP" ("SMS controls")
                        # "preparing HULK SMS!"
                        # "actual sweep rate"
                        # "1sec delay\nbecause HULK is not very bright"
                        # "sets sweep rate for HULK SMS"
                        n191 = local read item#-1() -> (w148)
                        n192 = local read "Hulk_SMS_addr"() -> (w147:refnum<visa-resource-name>)
                        n193 = local read item#-1() -> (w145)
                        n194 = call "SweepRateConversion.vi"("RAMP rate in"=w148, "T/min to A/s (True)"=TRUE) -> ("RAMP rate out"=w146:dbl)
                        n195 = call "SMSsendCommand.vi"("HULK SMS address in"=w147, "SMS controls"=w134, "error in"=w145, "RAMP rate"=w146) -> ("HULK SMS address out"=w141:refnum<visa-resource-name>, "error out"=w142:errorcluster)  [unwired: 13 in, 1 out]
                        n196 = call "WaitRS232.vi"("error in"=w142, "delay[160 ms]"=u32 1000) -> ("error out"=w144:errorcluster)  [unwired: 1 in]
                        n197 = call "SMSread.vi"("HULK SMS address in"=w141, "SMS controls"=w134, "error in"=w144) -> ("read buffer"=w137:string, "error out"=w138:errorcluster)  [unwired: 11 in, 4 out]
                        n198 = Match Pattern(string=w137, regular expression="RAMP RATE:") -> (after substring=w140:string)  [unwired: 1 in, 3 out]
                        n199 = local write item#-1(w137) -> ()
                        n200 = Scan From String(format string="%.f", input string=w140, error in=w138) -> (error out=w135:errorcluster, output 1=w133:dbl)  [unwired: 2 in, 2 out]
                        n201 = local write item#-1(w135) -> ()
                        n202 = call "SweepRateConversion.vi"("RAMP rate in"=w133, "T/min to A/s (True)"=FALSE) -> ("RAMP rate out"=w131:dbl)
                        n203 = local write item#-1(w131) -> ()
                      }
                      frame #6 {
                        w150 = SMScontrols."SET MID" ("SMS controls")
                        # "sets target value for B field sweep"
                        n204 = local read "Hulk_SMS_addr"() -> (w153:refnum<visa-resource-name>)
                        n205 = local read item#-1() -> (w154)
                        n206 = local read item#-1() -> (w152)
                        n207 = call "SMSsendCommand.vi"("HULK SMS address in"=w153, "SMS controls"=w150, "error in"=w154, "MID field value"=w152) -> ("HULK SMS address out"=w158:refnum<visa-resource-name>, "error out"=w156:errorcluster)  [unwired: 13 in, 1 out]
                        n208 = call "WaitRS232.vi"("error in"=w156, "delay[160 ms]"=u32 1000) -> ("error out"=w157:errorcluster)  [unwired: 1 in]
                        n209 = call "SMSread.vi"("HULK SMS address in"=w158, "SMS controls"=w150, "error in"=w157) -> ("read buffer"=w151:string, "error out"=w155:errorcluster)  [unwired: 11 in, 4 out]
                        n210 = local write item#-1(w155) -> ()
                        n211 = local write item#-1(w151) -> ()
                      }
                      frame #7 {
                        # "acquires current output value"
                        n212 = local read "Hulk_SMS_addr"() -> (w164:refnum<visa-resource-name>)
                        n213 = local read item#-1() -> (w163)
                        n214 = call "SMS_GET_OUTPUT.vi"("CRYogenic:("=w163, "Hulk_SMS_addr"=w164) -> ("error IO"=w160:errorcluster, "read buffer"=w162:string, "Numeric"=w161:dbl)
                        n215 = local write item#-1(w160) -> ()
                        n216 = local write item#-1(w162) -> ()
                      }
                      frame #8 {
                        # "activates ramping"
                        n217 = local read item#-1() -> (w172)
                        n218 = Equal?(x=w172, y=0.0) -> (x = y?=w170:bool)
                        n219 = Select(t=SMScontrols."RAMP ZERO" ("SMS controls"), s=w170, f=SMScontrols."RAMP MID" ("SMS controls")) -> (s? t:f=w167:T12)
                        n220 = local read "Hulk_SMS_addr"() -> (w174:refnum<visa-resource-name>)
                        n221 = local read item#-1() -> (w173)
                        n222 = call "SMSsendCommand.vi"("HULK SMS address in"=w174, "SMS controls"=w167, "error in"=w173) -> ("HULK SMS address out"=w177:refnum<visa-resource-name>, "error out"=w176:errorcluster)  [unwired: 14 in, 1 out]
                        n223 = call "WaitRS232.vi"("error in"=w176, "delay[160 ms]"=u32 1000) -> ("error out"=w178:errorcluster)  [unwired: 1 in]
                        n224 = call "SMSread.vi"("HULK SMS address in"=w177, "SMS controls"=w167, "error in"=w178) -> ("read buffer"=w165:string, "error out"=w166:errorcluster)  [unwired: 11 in, 4 out]
                        n225 = local write item#-1(w166) -> ()
                        n226 = local write item#-1(w165) -> ()
                      }
                    }
                  }
                  frame Enabled {
                    # "preparing Teslatron_iPS_Field"
                    # "Measure magnetic field on Teslatron_iPS_Field"
                    n227 = property on="iPS_addr_sweep" class="VISAName"() -> ("Value"=w181:refnum<visa-resource-name>)  [unwired: 2 in, 2 out]
                    n228 = call "iPSread.vi"("iPSreadCtrl"=iPSreadCtrl."OutputField", "VISA resource name"=w181) -> ("number"=w180:dbl)  [unwired: 6 in, 3 out]
                  }
                }
              }
              frame "iTC" {
                n229 = disable-structure shown="Enabled" {
                  disable-tunnel: [w190 w195] -> w182
                  frame Disabled {
                    w193 = u16 0 items=["Volts", "Current", "Auto Resistance", "Manual Resistance", "Digitize Voltage", "Digitize Current"] ("Function (0: Volts)")
                    w187 = u16 1 items=["Volts", "Current"] ("Function (0: Volts)")
                    n230 = call <instrlib>:"Configure Source Limit Level.vi"("Source Limit (1.0)"=5.0, "Function (0: Volts)"=w187) -> ("error out"=w185:errorcluster, "VISA resource name out"=w188:refnum<visa-resource-name>, "VISA resource name"=w189:refnum<visa-resource-name>)  [unwired: 7 in]
                    n231 = call <instrlib>:"Configure Measurement Function.vi"("error in (no error)"=w185, "Function (0: Volts)"=w193, "VISA resource name"=w188) -> ("error out"=w184:errorcluster, "VISA resource name out"=w192:refnum<visa-resource-name>)  [unwired: 7 in]
                    n232 = call <instrlib>:"Enable Output.vi"("error in (no error)"=w184, "VISA resource name"=w192) -> ("error out"=w183:errorcluster, "VISA resource name out"=w191:refnum<visa-resource-name>)  [unwired: 8 in]
                    n233 = call <instrlib>:"Get Source Level.vi"("error in (no error)"=w183, "VISA resource name"=w191) -> ("Current Level Out"=w190:dbl)  [unwired: 6 in, 3 out]
                  }
                  frame Enabled {
                    n234 = property on="iPS_addr_sweep" class="VISAName"() -> ("Value"=w194:refnum<visa-resource-name>)  [unwired: 2 in, 2 out]
                    n235 = call "iTCread.vi"("VISA resource name"=w194, "iTCreadCtrl"=iTCreadCtrl."Sample Temp") -> ("number"=w195:dbl)  [unwired: 5 in, 3 out]
                  }
                }
              }
              frame "AuxOut0" {
                n236 = disable-structure shown="Disabled" {
                  disable-tunnel: [w200 0.0 ("AuxOut0_Ampl")] -> w197
                  frame Disabled {
                    n237 = property on="MFLI1_addr" class="Str"() -> ("Value"=w199:string)  [unwired: 2 in, 2 out]
                    n238 = call <instrlib>:"ziOpen.vi"("Address"=w199) -> ("HandleOut"=w198:T1)  [unwired: 3 in, 2 out]
                    n239 = property on="HandleOut" class="Clust (strict)"("Value"=w198) -> ()  [unwired: 2 in, 2 out]
                    n240 = call "MFLIcontrol.vi"("MFLI function"=MFLIcommand."Get AuxOut0", "handle in"=w198) -> ("AuxOut0_Ampl"=w200:dbl)  [unwired: 5 in, 4 out]
                  }
                  frame Enabled {
                  }
                }
              }
            }
            n241 = property on="Sweep Channel" class="DigNum (strict)"("Value"=w63) -> ()  [unwired: 2 in, 2 out]
          }
          frame #1 {
            # "Read Current value of step channel"
            n242 = property on="Linetrace or Mapping?" class="Bool (strict)"() -> ("Value"=w203:bool)  [unwired: 2 in, 2 out]
            n243 = case shown="True" w203 {
              frame False {
                w204 = 9999999.0 ("Step Channel")
                n244 = property on="Step Channel" class="DigNum (strict)"("Value"=w204) -> ()  [unwired: 2 in, 2 out]
                n245 = property on="Hyper Channel" class="DigNum (strict)"("Value"=w204) -> ()  [unwired: 2 in, 2 out]
              }
              frame True {
                # "1 = 2400 1\n2 = 2400 2\n3 = 2400 3\n4 = 2636a smua\n5 = 2636a smub\n6 = do not sweep, just time\n7 =IPS120-10\n8 =2461_smu"
                n246 = property on="step" class="RadioBtnsControl (strict)"() -> ("Value"=w206:T5)  [unwired: 2 in, 2 out]
                n247 = case "reads current value from instrument which will be sweeping" shown="\"2636_smub_step\"" w206 {
                  tunnel: [w208 w218 w227 w231 0.0 ("Measuremet") w237 w238 w239] -> w205
                  frame "V2400_1_Step", Default {
                    # "reads the voltage on 2400 1"
                    n248 = property on="2400_1_addr_step" class="DigNum (strict)"() -> ("Value"=w207:u8)  [unwired: 2 in, 2 out]
                    n249 = Number To Decimal String(number=w207) -> (decimal integer string=w212:string)  [unwired: 1 in]
                    n250 = GPIB Write(0:w212, 1:":READ?") -> (6:w209:errorcluster)  [unwired: 3 in, 1 out]
                    n251 = GPIB Read(0:w212, 1:3200, 3:w209) -> (5:w214:string)  [unwired: 2 in, 2 out]
                    n252 = String Subset(string=w214, length (rest)=13) -> (substring=w215:string)  [unwired: 1 in]
                    n253 = Fract/Exp String To Number(string=w215) -> (number=w208:dbl)  [unwired: 3 in, 1 out]
                  }
                  frame "V2400_2_step" {
                    # "reads the current on 2400 2"
                    n254 = property on="2400_2_addr_step" class="DigNum (strict)"() -> ("Value"=w216:u8)  [unwired: 2 in, 2 out]
                    n255 = Number To Decimal String(number=w216) -> (decimal integer string=w222:string)  [unwired: 1 in]
                    n256 = GPIB Write(0:w222, 1:":READ?") -> (6:w219:errorcluster)  [unwired: 3 in, 1 out]
                    n257 = GPIB Read(0:w222, 1:3200, 3:w219) -> (5:w224:string)  [unwired: 2 in, 2 out]
                    n258 = String Subset(string=w224, offset (0)=14, length (rest)=13) -> (substring=w225:string)
                    n259 = Fract/Exp String To Number(string=w225) -> (number=w218:dbl)  [unwired: 3 in, 1 out]
                  }
                  frame "2636_smua_step" {
                    # "reads the voltage on 2636a smua"
                    n260 = property on="2614A_addr_step" class="VISAName"() -> ("Value"=w226:refnum<visa-resource-name>)  [unwired: 2 in, 2 out]
                    n261 = call "SinglePointMeasurement.vi"("Measure"=Measure."Voltage", "Channel"=Channel."a", "VISA resource name 2"=w226) -> ("Measuremet"=w227:dbl)  [unwired: 3 in, 4 out]
                  }
                  frame "2636_smub_step" {
                    # "reads the voltage on 2636a smub"
                    n262 = property on="2614A_addr_step" class="VISAName"() -> ("Value"=w230:refnum<visa-resource-name>)  [unwired: 2 in, 2 out]
                    n263 = call "SinglePointMeasurement.vi"("Measure"=Measure."Voltage", "Channel"=Channel."b", "VISA resource name 2"=w230) -> ("Measuremet"=w231:dbl)  [unwired: 3 in, 4 out]
                  }
                  frame "time_step" {
                  }
                  frame "iPS_step" {
                    # "Measure magnetic field on IPS"
                    n264 = property on="iPS _addr_step" class="VISAName"() -> ("Value"=w236:refnum<visa-resource-name>)  [unwired: 2 in, 2 out]
                    n265 = call "iPSread.vi"("iPSreadCtrl"=iPSreadCtrl."OutputField", "VISA resource name"=w236) -> ("number"=w237:dbl)  [unwired: 6 in, 3 out]
                  }
                  frame "iTC_step" {
                    n266 = call "TRITON_Read Temperature.vi"() -> ("Measuremet"=w238:dbl)  [unwired: 2 in, 1 out]
                  }
                  frame "2461_Curr" {
                    n267 = property on="2461_addr_sweep" class="VISAName"() -> ("Value"=w240:refnum<visa-resource-name>)  [unwired: 2 in, 2 out]
                    n268 = call <instrlib>:"Get Source Level.vi"("VISA resource name"=w240) -> ("Current Level Out"=w239:dbl)  [unwired: 7 in, 3 out]
                  }
                }
                n269 = property on="Step Channel" class="DigNum (strict)"("Value"=w205) -> ()  [unwired: 2 in, 2 out]
              }
            }
          }
          frame #2 {
            # "Read Current value of hyp[er loop channel"
            n270 = property on="HyperLoop" class="Bool (strict)"() -> ("Value"=w241:bool)  [unwired: 2 in, 2 out]
            n271 = case shown="True" w241 {
              frame False {
                n272 = property on="Hyper Channel" class="DigNum (strict)"("Value"=9999999.0 ("Step Channel")) -> ()  [unwired: 2 in, 2 out]
              }
              frame True {
                # "1 = 2400 1\n2 = 2400 2\n3 = 2400 3\n4 = 2636a smua\n5 = 2636a smub\n6 = do not sweep, just time\n7 =IPS120-10\n8 =2461_smu"
                n273 = property on="step_hyper" class="RadioBtnsControl (strict)"() -> ("Value"=w244:T6)  [unwired: 2 in, 2 out]
                n274 = case "reads current value from instrument which will be sweeping" shown="\"iTC_HyperLoop\"" w244 {
                  tunnel: [w246 w256 w265 w269 0.0 ("Measuremet") w275 w277] -> w243
                  frame "2400_1_HyperLoop", Default {
                    # "reads the voltage on 2400 1"
                    n275 = property on="2400_1_addr_hyper" class="DigNum (strict)"() -> ("Value"=w245:u8)  [unwired: 2 in, 2 out]
                    n276 = Number To Decimal String(number=w245) -> (decimal integer string=w250:string)  [unwired: 1 in]
                    n277 = GPIB Write(0:w250, 1:":READ?") -> (6:w247:errorcluster)  [unwired: 3 in, 1 out]
                    n278 = GPIB Read(0:w250, 1:3200, 3:w247) -> (5:w252:string)  [unwired: 2 in, 2 out]
                    n279 = String Subset(string=w252, length (rest)=13) -> (substring=w253:string)  [unwired: 1 in]
                    n280 = Fract/Exp String To Number(string=w253) -> (number=w246:dbl)  [unwired: 3 in, 1 out]
                  }
                  frame "2400_2_HyperLoop" {
                    # "reads the current on 2400 2"
                    n281 = property on="2400_2_addr_hyper" class="DigNum (strict)"() -> ("Value"=w254:u8)  [unwired: 2 in, 2 out]
                    n282 = Number To Decimal String(number=w254) -> (decimal integer string=w260:string)  [unwired: 1 in]
                    n283 = GPIB Write(0:w260, 1:":READ?") -> (6:w257:errorcluster)  [unwired: 3 in, 1 out]
                    n284 = GPIB Read(0:w260, 1:3200, 3:w257) -> (5:w262:string)  [unwired: 2 in, 2 out]
                    n285 = String Subset(string=w262, offset (0)=14, length (rest)=13) -> (substring=w263:string)
                    n286 = Fract/Exp String To Number(string=w263) -> (number=w256:dbl)  [unwired: 3 in, 1 out]
                  }
                  frame "2636_smua_HyperLoop" {
                    # "reads the voltage on 2636a smua"
                    n287 = property on="2336A_addr_hyper" class="VISAName"() -> ("Value"=w264:refnum<visa-resource-name>)  [unwired: 2 in, 2 out]
                    n288 = call "SinglePointMeasurement.vi"("Measure"=Measure."Voltage", "Channel"=Channel."a", "VISA resource name 2"=w264) -> ("Measuremet"=w265:dbl)  [unwired: 3 in, 4 out]
                  }
                  frame "2636_smub_HyperLoop" {
                    # "reads the voltage on 2636a smub"
                    n289 = property on="2336A_addr_hyper" class="VISAName"() -> ("Value"=w268:refnum<visa-resource-name>)  [unwired: 2 in, 2 out]
                    n290 = call "SinglePointMeasurement.vi"("Measure"=Measure."Voltage", "Channel"=Channel."b", "VISA resource name 2"=w268) -> ("Measuremet"=w269:dbl)  [unwired: 3 in, 4 out]
                  }
                  frame "time_HyperLoop" {
                  }
                  frame "iPS_HyperLoop" {
                    # "Measure magnetic field on IPS"
                    n291 = property on="iPS _addr_hyper" class="VISAName"() -> ("Value"=w273:refnum<visa-resource-name>)  [unwired: 2 in, 2 out]
                    n292 = call "iPSread.vi"("iPSreadCtrl"=iPSreadCtrl."OutputField", "VISA resource name"=w273) -> ("number"=w275:dbl)  [unwired: 6 in, 3 out]
                  }
                  frame "iTC_HyperLoop" {
